vi "class discovery singleton.vi"(6 "Folders to Exclude":string[](array[string]), 8 "error in":errorcluster, 9 "Plugin Search Paths":path[](array[path]), 10 "Class Name":string, 11 "method":T1) -> (0 "error out":errorcluster, 1 "class path":path, 2 "LabVIEW Object":refnum<class>, 4 "discovered classes":path[](array[path]))   [LabVIEW 2013, in "class discovery singleton.lvlib"]
doc: "A functional global variable which provides name-based lookup of classes. When a search path is added, the FGV will locate all classes on disk and use the *filename* to cache them in memory. That is, the class c:\\classes\\foo.lvclass is stored as foo, not as FrameworkClasses.lvlib::Foo.lvclass. The assumption is that anything already in memory can be loaded by other means. When a load is requested, the FGV will first use the name as an input to get lvclass default value by name (which does expect FrameworkClasses.lvlib::Foo.lvclass). Then it will look for foo.lvclass in the list of found classes on disk. Then if all else fails, it will attempt to match a class in memory using a string match."
uses:
  class discovery singleton.lvlib
  class discovery singleton methods.ctl
  NISE_CEF_TreeControl.lvlib
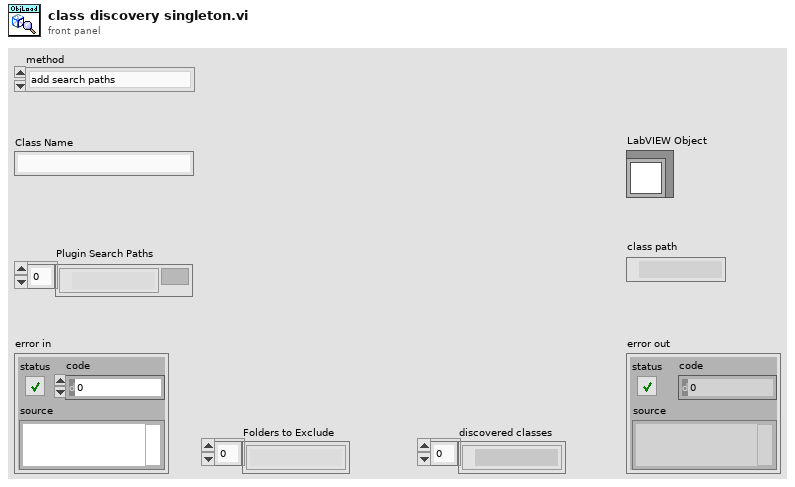
[diagram p1: front panel]
types:
  T1 = typedef "class discovery singleton.lvlib/class discovery singleton methods.ctl" = enum16{"add search paths", "load class by name", "list available classes", "get class path"}
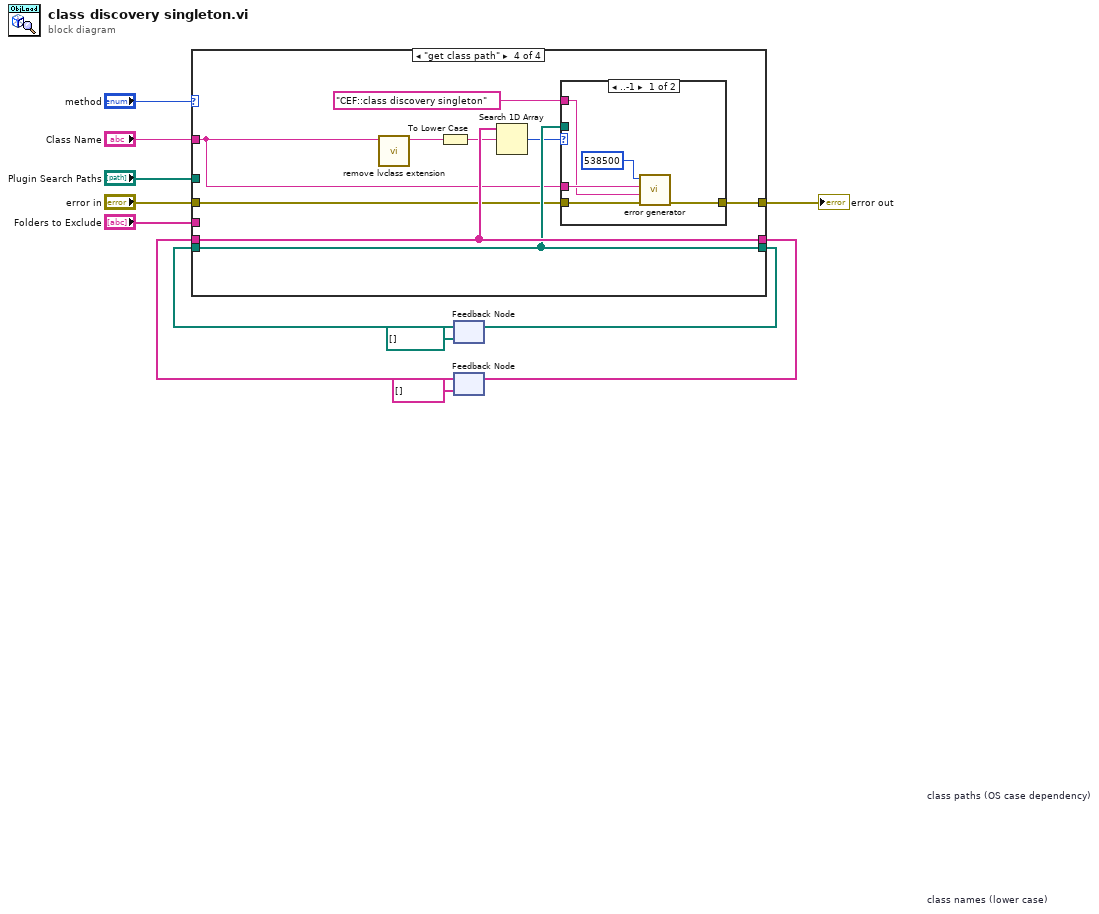
[diagram p0: block diagram]
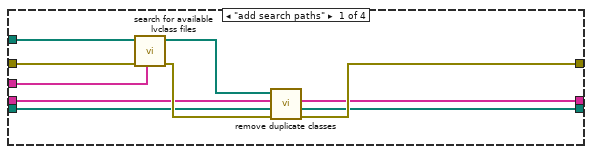
[diagram p2: hidden frame]
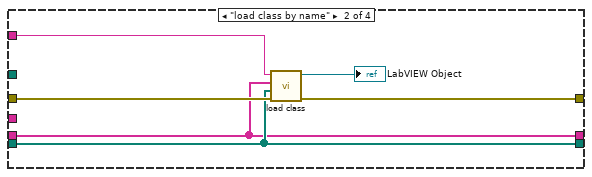
[diagram p3: hidden frame]
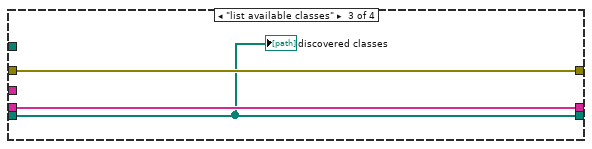
[diagram p4: hidden frame]
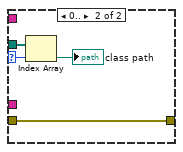
[diagram p5: hidden frame]
diagram:
  n1 = feedback #1 "class paths (OS case dependency)"(path[] [] ("class paths out")) -> (w5:path[])
  n2 = feedback #2 "class names (lower case)"(string[] [] ("class names out")) -> (w7:string[])
  n3 = case shown="\"get class path\"" "method" {
    tunnel: "error in" -> [w22 w28 w30 w37]
    tunnel: "Plugin Search Paths" -> [w21 _ _ _]
    tunnel: [w18 w27 w30 w36] -> w9
    tunnel: w7 -> [w17 w25 w31 w40]
    tunnel: [w16 w25 w31 w40] -> w8
    tunnel: [w15 w26 w29 w39] -> w6
    tunnel: w5 -> [w14 w26 w29 w39]
    tunnel: "Class Name" -> [_ w24 _ w35]
    tunnel: "Folders to Exclude" -> [w13 _ _ _]
    frame "add search paths" {
      n4 = call "search for available lvclass files.vi"("Folders to Exclude"=w13, "error in"=w22, "Plugin Search Paths"=w21) -> ("error out"=w19:errorcluster, "discovered classes"=w20:path[])  [unwired: 7 in]
      n5 = call "remove duplicate classes.vi"("error in"=w19, "class paths in"=w14, "class names in"=w17, "discovered classes"=w20) -> ("error out"=w18:errorcluster, "class paths out"=w15:path[], "class names out"=w16:string[])  [unwired: 5 in]
    }
    frame "load class by name" {
      n6 = call "load class.vi"("error in"=w28, "available class paths"=w26, "available class names"=w25, "Class Name"=w24) -> ("error out"=w27:errorcluster, "Object Out"=→"LabVIEW Object":refnum<class>)  [unwired: 6 in]
    }
    frame "list available classes" {
      "discovered classes" <- w29
    }
    frame "get class path" {
      n7 = call "remove lvclass extension.vi"("class name in"=w35) -> ("class name out"=w34:string)  [unwired: 10 in]
      n8 = To Lower Case(string=w34) -> (all lower case string=w33:string)
      n9 = Search 1D Array(1D array=w40, element=w33) -> (index of element=w38:i32)  [unwired: 1 in]
      n10 = case shown="..-1" w38 {
        selector: w38 -> [_ w48]
        tunnel: w39 -> [_ w49]
        tunnel: w37 -> [w44 w47]
        tunnel: [w45 w47] -> w36
        tunnel: w35 -> [w43 _]
        tunnel: "CEF::class discovery singleton" -> [w41 _]
        frame ..-1 {
          n11 = call "error generator.vi"("error in"=w44, "source"=w41, "append error message"=w43, "error code (0)"=538500) -> ("error out"=w45:errorcluster)  [unwired: 5 in]
        }
        frame 0.. {
          n12 = Index Array(array=w49, index=w48) -> (element=→"class path":path)
        }
      }
    }
  }
  "error out" <- w9
  n13 = feedback-in #1(w6) -> ()
  n14 = feedback-in #2(w8) -> ()
